vi "Frequency Control Master Table.vi"() -> (1 "Sample Rate":dbl[](array[numeric]), 2 "Frequency":dbl[](array[numeric]), 3 "Table Index":dbl[](array[numeric]))   [LabVIEW 2010]
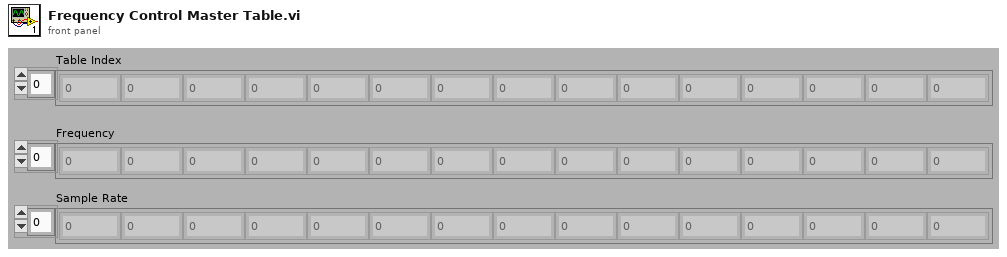
[diagram p1: front panel]
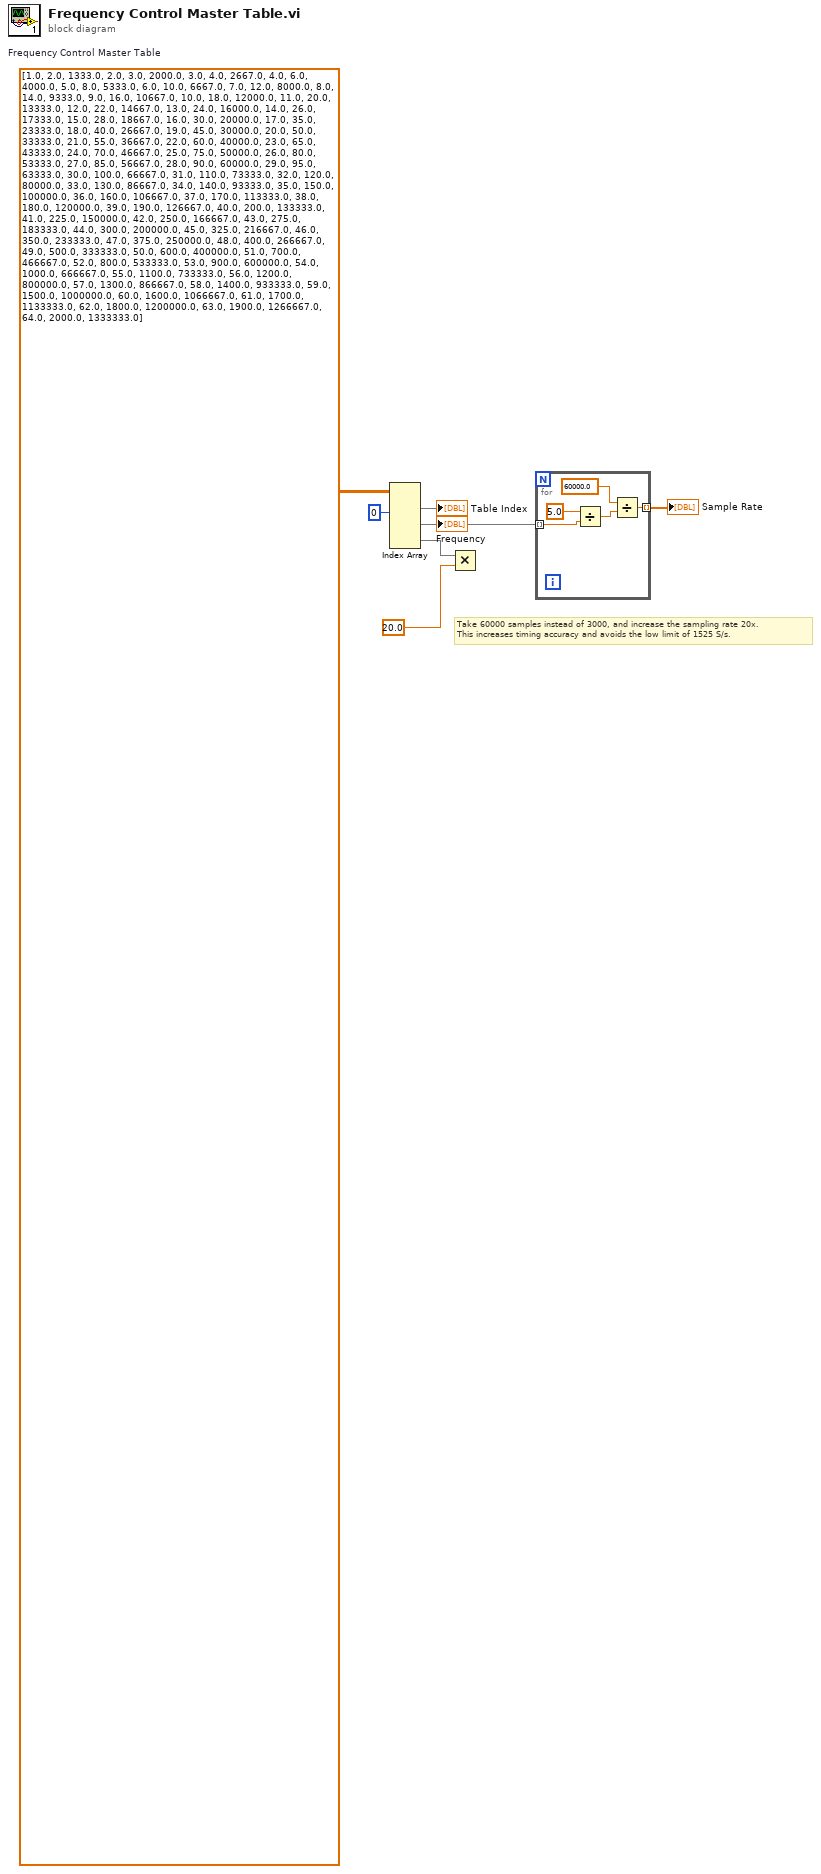
[diagram p0: block diagram]
diagram:
  w7 = dbl[][] [[1.0, 2.0, 1333.0], [2.0, 3.0, 2000.0], [3.0, 4.0, 2667.0], [4.0, 6.0, 4000.0], [5.0, 8.0, 5333.0], [6.0, 10.0, 6667.0], [7.0, 12.0, 8000.0], [8.0, 14.0, 9333.0], [9.0, 16.0, 10667.0], [10.0, 18.0, 12000.0], [11.0, 20.0, 13333.0], [12.0, 22.0, 14667.0], [13.0, 24.0, 16000.0], [14.0, 26.0, 17333.0], [15.0, 28.0, 18667.0], [16.0, 30.0, 20000.0], [17.0, 35.0, 23333.0], [18.0, 40.0, 26667.0], [19.0, 45.0, 30000.0], [20.0, 50.0, 33333.0], [21.0, 55.0, 36667.0], [22.0, 60.0, 40000.0], [23.0, 65.0, 43333.0], [24.0, 70.0, 46667.0], [25.0, 75.0, 50000.0], [26.0, 80.0, 53333.0], [27.0, 85.0, 56667.0], [28.0, 90.0, 60000.0], [29.0, 95.0, 63333.0], [30.0, 100.0, 66667.0], [31.0, 110.0, 73333.0], [32.0, 120.0, 80000.0], [33.0, 130.0, 86667.0], [34.0, 140.0, 93333.0], [35.0, 150.0, 100000.0], [36.0, 160.0, 106667.0], [37.0, 170.0, 113333.0], [38.0, 180.0, 120000.0], [39.0, 190.0, 126667.0], [40.0, 200.0, 133333.0], [41.0, 225.0, 150000.0], [42.0, 250.0, 166667.0], [43.0, 275.0, 183333.0], [44.0, 300.0, 200000.0], [45.0, 325.0, 216667.0], [46.0, 350.0, 233333.0], [47.0, 375.0, 250000.0], [48.0, 400.0, 266667.0], [49.0, 500.0, 333333.0], [50.0, 600.0, 400000.0], [51.0, 700.0, 466667.0], [52.0, 800.0, 533333.0], [53.0, 900.0, 600000.0], [54.0, 1000.0, 666667.0], [55.0, 1100.0, 733333.0], [56.0, 1200.0, 800000.0], [57.0, 1300.0, 866667.0], [58.0, 1400.0, 933333.0], [59.0, 1500.0, 1000000.0], [60.0, 1600.0, 1066667.0], [61.0, 1700.0, 1133333.0], [62.0, 1800.0, 1200000.0], [63.0, 1900.0, 1266667.0], [64.0, 2000.0, 1333333.0]]  # Frequency Control Master Table
  # "Take 60000 samples instead of 3000, and increase the sampling rate 20x.\nThis increases timing accuracy and avoids the low limit of 1525 S/s."
  n1 = Index Array(array=w7, index (col) #1=0 ("disabled index (col)")) -> (element #1=→"Table Index":dbl[], element #2=w2:dbl[], element #3=w4:dbl[])  [unwired: 5 in]
  "Frequency" <- w2
  n2 = Multiply(x=w4, y=20.0) -> ()  [unwired: 1 out]
  n3 = for {
    tunnel: w2 -> [w12] mode=indexing
    tunnel: [w8] -> w1 mode=indexing
    n4 = Divide(x=5.0, y=w12) -> (x/y=w9:dbl)
    n5 = Divide(x=60000.0, y=w9) -> (x/y=w8:dbl)
  }
  "Sample Rate" <- w1
